vi "DAQ.Read.vi"(8 "error in (no error)":errorcluster, 11 "DAQ in":refnum<class "DAQ.lvclass">) -> (0 "error out":errorcluster, 2 "Read":waveform(dbl)[](array[waveform]), 3 "DAQ out":refnum<class "DAQ.lvclass">)   [LabVIEW 2020, in "DAQ.lvclass"]
uses:
  DAQ.lvclass
  DAQ.lvclass/DAQ.ctl
  <vilib>/measure/NI_MABase.lvlib
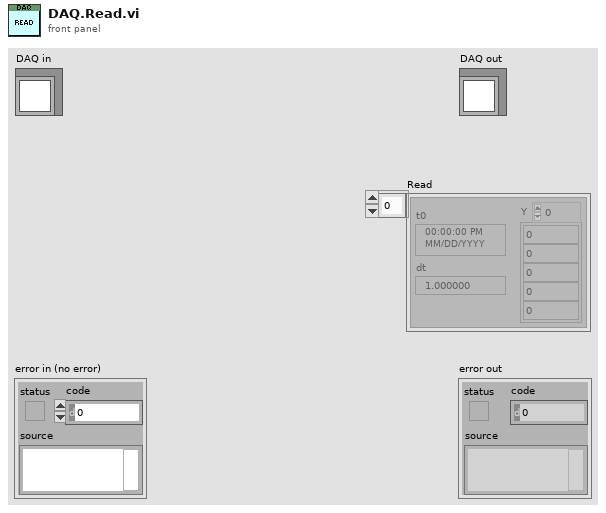
[diagram p1: front panel]
types:
  T1 = typedef "DAQ.lvclass/DAQ_SamplingInfo.ctl" = cluster{"Fs":dbl, "#s":i32}
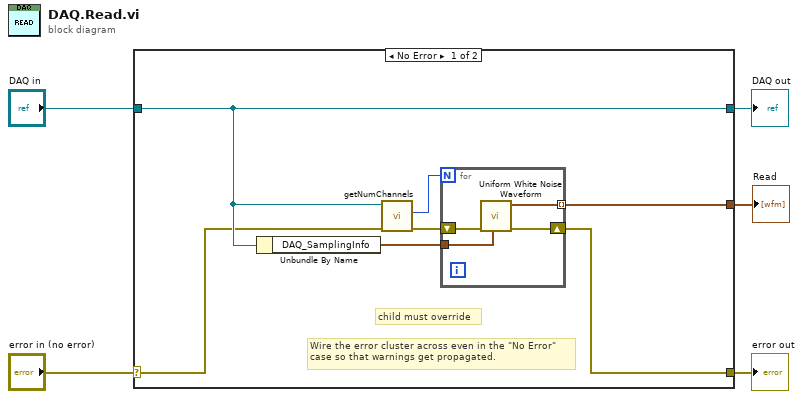
[diagram p0: block diagram]
diagram:
  n1 = case shown="No Error" "error in (no error)" {
    selector: "error in (no error)" -> [w7 w18]
    tunnel: [w6 w18] -> w4
    tunnel: [w10 w17] -> w2
    tunnel: "DAQ in" -> [w10 w17]
    tunnel: [w12 _] -> w1
    frame No Error {
      # "child must override"
      # "Wire the error cluster across even in the \"No Error\"\ncase so that warnings get propagated."
      n2 = Unbundle By Name(w10) -> ("DAQ_SamplingInfo"=w9:T1)
      n3 = call "getNumChannels.vi"("error in (no error)"=w7, "DAQ in"=w10) -> ("error out"=w8:errorcluster, "NumChannels"=w11:i32)  [unwired: 7 in, 1 out]
      n4 = for {
        N: w11 -> [_]
        tunnel: [w16] -> w12 mode=indexing
        tunnel: w9 -> [w15]
        shift-right: [w13] -> w6
        shift-left: w8 -> [w14]
        n5 = call <vilib>:"Uniform White Noise Waveform.vi"("sampling info"=w15, "error in (no error)"=w14) -> ("error out"=w13:errorcluster, "signal out"=w16:waveform(dbl))  [unwired: 8 in]
      }
    }
    frame Error {
    }
  }
  "error out" <- w4
  "DAQ out" <- w2
  "Read" <- w1
